vi "Read Test.vi"(8 "error in (no error)":errorcluster, 9 "data table":T1, 10 "data dictionary":refnum<class "data dictionary.lvclass">, 11 "runtime in":refnum<class "SystemLink File runtime.lvclass">) -> (0 "error out":errorcluster, 2 "Pass":bool[](array[boolean]), 3 "runtime out":refnum<class "SystemLink File runtime.lvclass">)   [LabVIEW 2015, in "SystemLink File Module tests.lvlib"]
uses:
  SystemLink File Module tests.lvlib
  <vilib>/NI/Tag Bus/dictionary/data dictionary.lvclass
  <vilib>/NI/Tag Bus/dictionary/lookup polymorphs/locate double.vi
  module/execution/SystemLink File runtime.lvclass
  <vilib>/NI/Tag Bus/table/data table.lvlib
  <vilib>/NI/Tag Bus/table/data polymorphs/read one/read Double.vi
  <vilib>/Skyline/Tag/Wrapper/Wrapper_class/NI Skyline Tag.lvclass
  <vilib>/Skyline/Tag/Wrapper/Wrapper AMQP_class/Open Tag AMQP.vi
  <vilib>/Skyline/Tag/Wrapper/Wrapper AMQP_class/NI Skyline Tag AMQP.lvclass
  <vilib>/Skyline/Tag/Wrapper/Wrapper_class/Write Tag (DBL).vi
  <vilib>/Skyline/Tag/Wrapper/Wrapper_class/Close Tag (Single).vi
  <vilib>/Skyline/Tag/Wrapper/Wrapper_class/Write Tag (I32).vi
  <vilib>/Skyline/Tag/Wrapper/Wrapper_class/Write Tag (String).vi
  <vilib>/NI/Tag Bus/table/data polymorphs/read one/read I32.vi
  <vilib>/NI/Tag Bus/dictionary/lookup polymorphs/locate I32.vi
  <vilib>/Skyline/Tag/Wrapper/Wrapper_class/Write Tag (U64).vi
  <vilib>/Skyline/Tag/Wrapper/Wrapper_class/Write Tag (Boolean).vi
  module/configuration/SystemLink File configuration.lvclass
  <vilib>/Skyline/Tag/Wrapper/Wrapper_class/Write Tag (Timestamp).vi
  <vilib>/NI/Tag Bus/dictionary/lookup polymorphs/locate Single.vi
  <vilib>/NI/Tag Bus/table/data polymorphs/read one/read Single.vi
  <vilib>/NI/Tag Bus/dictionary/lookup polymorphs/locate I16.vi
  <vilib>/NI/Tag Bus/table/data polymorphs/read one/read I16.vi
  <vilib>/NI/Tag Bus/dictionary/lookup polymorphs/locate I8.vi
  <vilib>/NI/Tag Bus/table/data polymorphs/read one/read I8.vi
  <vilib>/NI/Tag Bus/dictionary/lookup polymorphs/locate U64.vi
  <vilib>/NI/Tag Bus/table/data polymorphs/read one/read U64.vi
  <vilib>/NI/Tag Bus/dictionary/lookup polymorphs/locate U32.vi
  <vilib>/NI/Tag Bus/table/data polymorphs/read one/read U32.vi
  <vilib>/NI/Tag Bus/dictionary/lookup polymorphs/locate U16.vi
  <vilib>/NI/Tag Bus/table/data polymorphs/read one/read U16.vi
  <vilib>/NI/Tag Bus/dictionary/lookup polymorphs/locate U8.vi
  <vilib>/NI/Tag Bus/table/data polymorphs/read one/read U8.vi
  <vilib>/NI/Tag Bus/dictionary/lookup polymorphs/locate Boolean.vi
  <vilib>/NI/Tag Bus/table/data polymorphs/read one/read Boolean.vi
  <vilib>/NI/Tag Bus/dictionary/lookup polymorphs/locate String.vi
  <vilib>/NI/Tag Bus/table/data polymorphs/read one/read String.vi
  <vilib>/NI/Tag Bus/table/data table.ctl
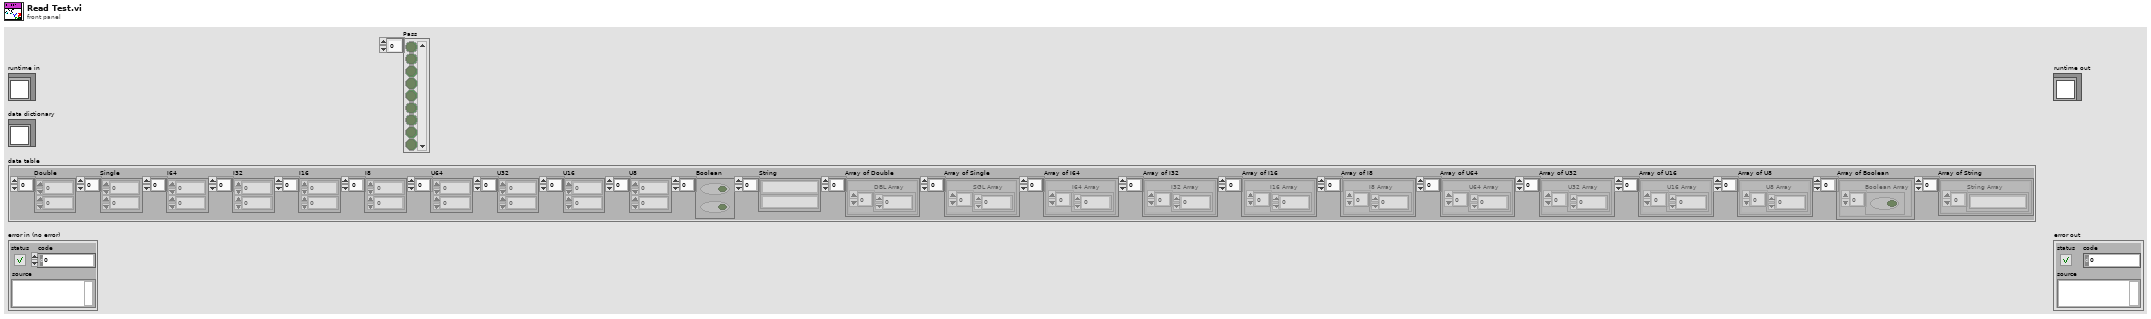
[diagram p1: front panel]
types:
  T1 = typedef "tag bus.lvlib/data table.lvlib/data table.ctl" = cluster{"Double":dbl[], "Single":sgl[], "I64":i64[], "I32":i32[], "I16":i16[], "I8":i8[], "U64":u64[], "U32":u32[], "U16":u16[], "U8":u8[], "Boolean":bool[], "String":string[], "Array of Double":cluster{"DBL Array":dbl[]}[], "Array of Single":cluster{"SGL Array":sgl[]}[], "Array of I64":cluster{"I64 Array":i64[]}[], "Array of I32":cluster{"I32 Array":i32[]}[], "Array of I16":cluster{"I16 Array":i16[]}[], "Array of I8":cluster{"I8 Array":i8[]}[], "Array of U64":cluster{"U64 Array":u64[]}[], "Array of U32":cluster{"U32 Array":u32[]}[], "Array of U16":cluster{"U16 Array":u16[]}[], "Array of U8":cluster{"U8 Array":u8[]}[], "Array of Boolean":cluster{"Boolean Array":bool[]}[], "Array of String":cluster{"String Array":string[]}[]}
  T2 = typedef "SystemLink File configuration.lvclass/SysLink Mapping.ctl" = cluster{"Data Type":T3, "Tag Reference":refnum<class "NI Skyline Tag.lvclass">, "Tag Bus Index":i32, "AMQP":bool, "Skylink Index":i32}
  T3 = typedef "SystemLink File configuration.lvclass/Data Tag Type.ctl" = enum16{"Double", "Single", "I32", "I16", "I8", "U64", "U32", "U16", "U8", "Boolean", "String", "Timestamp"}
  T4 = typedef "NI Skyline Tag.lvlib/DataType.ctl" = enum32{"Double", "I32", "String", "Boolean", "U64", "Timestamp"}
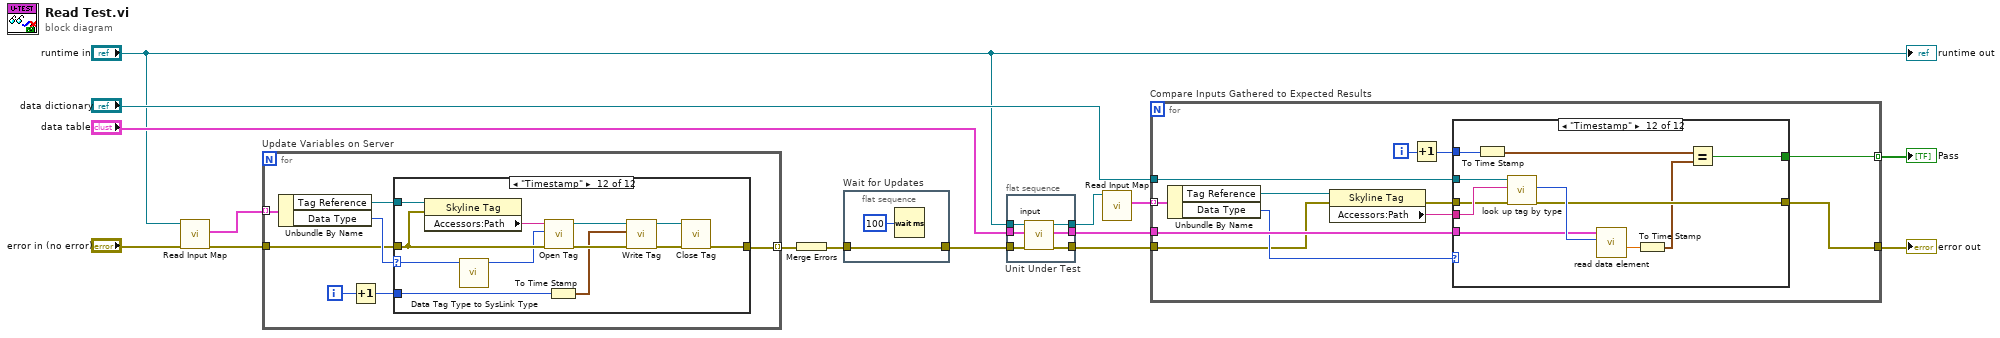
[diagram p0: block diagram]
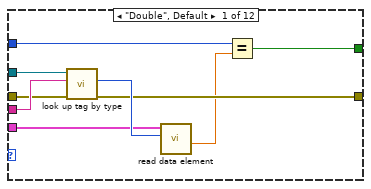
[diagram p2: hidden frame]
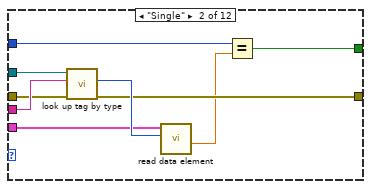
[diagram p3: hidden frame]
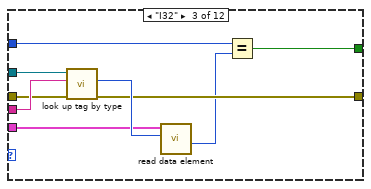
[diagram p4: hidden frame]
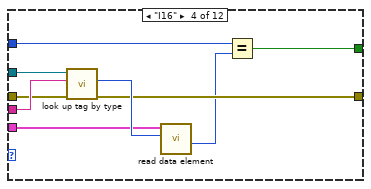
[diagram p5: hidden frame]
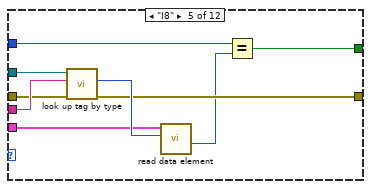
[diagram p6: hidden frame]
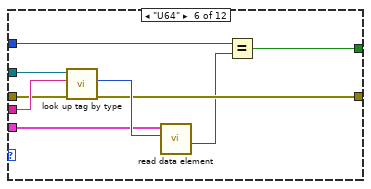
[diagram p7: hidden frame]
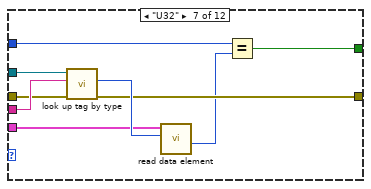
[diagram p8: hidden frame]
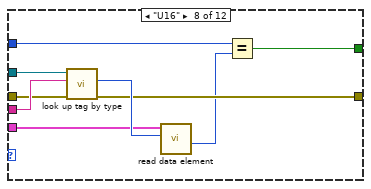
[diagram p9: hidden frame]
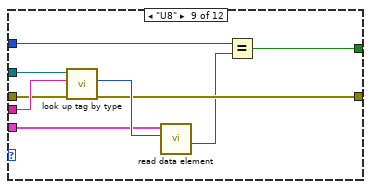
[diagram p10: hidden frame]
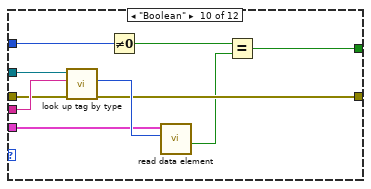
[diagram p11: hidden frame]
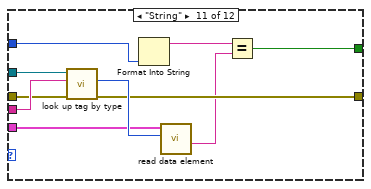
[diagram p12: hidden frame]
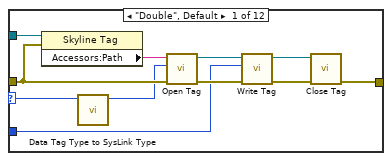
[diagram p13: hidden frame]
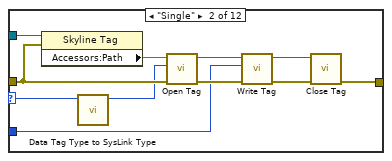
[diagram p14: hidden frame]
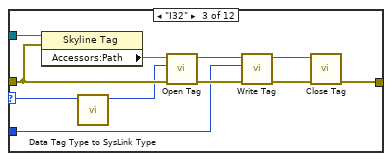
[diagram p15: hidden frame]
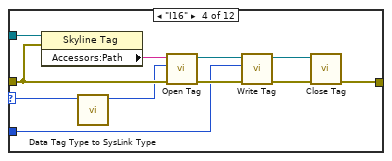
[diagram p16: hidden frame]
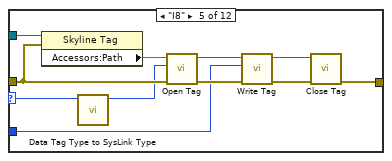
[diagram p17: hidden frame]
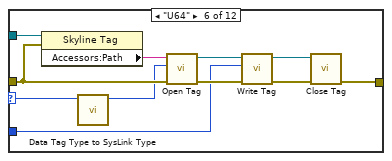
[diagram p18: hidden frame]
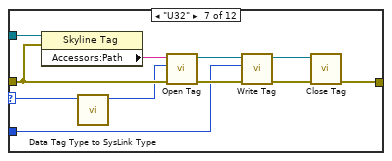
[diagram p19: hidden frame]
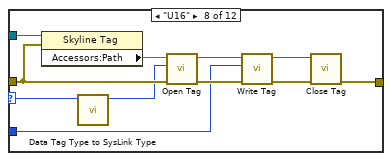
[diagram p20: hidden frame]
diagram:
  n1 = call "Read Input Map.vi"("error in (no error)"="error in (no error)", "SystemLink runtime in"="runtime in") -> ("error out"=w14:errorcluster, "Input Map"=w15:T2[])  [unwired: 7 in, 1 out]
  n2 = for "Update Variables on Server" {
    tunnel: w15 -> [w22] mode=indexing
    tunnel: w14 -> [w19]
    tunnel: [w16] -> w13 mode=indexing
    i -> [w18]
    n3 = Unbundle By Name(w22) -> ("Tag Reference"=w20:refnum<class "NI Skyline Tag.lvclass">, "Data Type"=w21:T3)
    n4 = Increment(x=w18) -> (x+1=w17:i32)
    n5 = case shown="\"Timestamp\"" w21 {
      selector: w21 -> [w30 w41 w52 w63 w74 w85 w96 w107 w118 w130 w142 w154]
      tunnel: w20 -> [w33 w44 w55 w66 w77 w88 w99 w110 w121 w133 w145 w157]
      tunnel: w19 -> [w31 w42 w53 w64 w75 w86 w97 w108 w119 w131 w143 w155]
      tunnel: w17 -> [w26 w37 w48 w59 w70 w81 w92 w103 w114 w126 w135 w147]
      tunnel: [w23 w34 w45 w56 w67 w78 w89 w100 w111 w123 w136 w148] -> w16
      frame "Double", Default {
        n6 = property class="Skyline Tag"(reference=w33, error in=w31) -> ("Accessors:Path"=w32:string)  [unwired: 2 out]
        n7 = call "Data Tag Type to SysLink Type.vi"("Data Tag Type"=w30) -> ("data type"=w29:T4)  [unwired: 10 in]
        n8 = call-poly <vilib>:"Open Tag.vi"("error in (no error)"=w31, "data type"=w29, "path"=w32) -> ("error out"=w27:errorcluster, "tag out"=w28:refnum<class "NI Skyline Tag.lvclass">)  [unwired: 7 in]
        n9 = call-poly <vilib>:"Write Tag.vi"("error in (no error)"=w27, "value"=w26, "tag in"=w28) -> ("error out"=w24:errorcluster, "tag out"=w25:refnum<class "NI Skyline Tag.lvclass">)  [unwired: 7 in]
        n10 = call-poly <vilib>:"Close Tag.vi"("error in (no error)"=w24, "tag in"=w25) -> ("error out"=w23:errorcluster)  [unwired: 9 in]
      }
      frame "Single" {
        n11 = property class="Skyline Tag"(reference=w44, error in=w42) -> ("Accessors:Path"=w43:string)  [unwired: 2 out]
        n12 = call "Data Tag Type to SysLink Type.vi"("Data Tag Type"=w41) -> ("data type"=w40:T4)  [unwired: 10 in]
        n13 = call-poly <vilib>:"Open Tag.vi"("error in (no error)"=w42, "data type"=w40, "path"=w43) -> ("error out"=w38:errorcluster, "tag out"=w39:refnum<class "NI Skyline Tag.lvclass">)  [unwired: 7 in]
        n14 = call-poly <vilib>:"Write Tag.vi"("error in (no error)"=w38, "value"=w37, "tag in"=w39) -> ("error out"=w35:errorcluster, "tag out"=w36:refnum<class "NI Skyline Tag.lvclass">)  [unwired: 7 in]
        n15 = call-poly <vilib>:"Close Tag.vi"("error in (no error)"=w35, "tag in"=w36) -> ("error out"=w34:errorcluster)  [unwired: 9 in]
      }
      frame "I32" {
        n16 = property class="Skyline Tag"(reference=w55, error in=w53) -> ("Accessors:Path"=w54:string)  [unwired: 2 out]
        n17 = call "Data Tag Type to SysLink Type.vi"("Data Tag Type"=w52) -> ("data type"=w51:T4)  [unwired: 10 in]
        n18 = call-poly <vilib>:"Open Tag.vi"("error in (no error)"=w53, "data type"=w51, "path"=w54) -> ("error out"=w49:errorcluster, "tag out"=w50:refnum<class "NI Skyline Tag.lvclass">)  [unwired: 7 in]
        n19 = call-poly <vilib>:"Write Tag.vi"("error in (no error)"=w49, "value"=w48, "tag in"=w50) -> ("error out"=w46:errorcluster, "tag out"=w47:refnum<class "NI Skyline Tag.lvclass">)  [unwired: 7 in]
        n20 = call-poly <vilib>:"Close Tag.vi"("error in (no error)"=w46, "tag in"=w47) -> ("error out"=w45:errorcluster)  [unwired: 9 in]
      }
      frame "I16" {
        n21 = property class="Skyline Tag"(reference=w66, error in=w64) -> ("Accessors:Path"=w65:string)  [unwired: 2 out]
        n22 = call "Data Tag Type to SysLink Type.vi"("Data Tag Type"=w63) -> ("data type"=w62:T4)  [unwired: 10 in]
        n23 = call-poly <vilib>:"Open Tag.vi"("error in (no error)"=w64, "data type"=w62, "path"=w65) -> ("error out"=w60:errorcluster, "tag out"=w61:refnum<class "NI Skyline Tag.lvclass">)  [unwired: 7 in]
        n24 = call-poly <vilib>:"Write Tag.vi"("error in (no error)"=w60, "value"=w59, "tag in"=w61) -> ("error out"=w57:errorcluster, "tag out"=w58:refnum<class "NI Skyline Tag.lvclass">)  [unwired: 7 in]
        n25 = call-poly <vilib>:"Close Tag.vi"("error in (no error)"=w57, "tag in"=w58) -> ("error out"=w56:errorcluster)  [unwired: 9 in]
      }
      frame "I8" {
        n26 = property class="Skyline Tag"(reference=w77, error in=w75) -> ("Accessors:Path"=w76:string)  [unwired: 2 out]
        n27 = call "Data Tag Type to SysLink Type.vi"("Data Tag Type"=w74) -> ("data type"=w73:T4)  [unwired: 10 in]
        n28 = call-poly <vilib>:"Open Tag.vi"("error in (no error)"=w75, "data type"=w73, "path"=w76) -> ("error out"=w71:errorcluster, "tag out"=w72:refnum<class "NI Skyline Tag.lvclass">)  [unwired: 7 in]
        n29 = call-poly <vilib>:"Write Tag.vi"("error in (no error)"=w71, "value"=w70, "tag in"=w72) -> ("error out"=w68:errorcluster, "tag out"=w69:refnum<class "NI Skyline Tag.lvclass">)  [unwired: 7 in]
        n30 = call-poly <vilib>:"Close Tag.vi"("error in (no error)"=w68, "tag in"=w69) -> ("error out"=w67:errorcluster)  [unwired: 9 in]
      }
      frame "U64" {
        n31 = property class="Skyline Tag"(reference=w88, error in=w86) -> ("Accessors:Path"=w87:string)  [unwired: 2 out]
        n32 = call "Data Tag Type to SysLink Type.vi"("Data Tag Type"=w85) -> ("data type"=w84:T4)  [unwired: 10 in]
        n33 = call-poly <vilib>:"Open Tag.vi"("error in (no error)"=w86, "data type"=w84, "path"=w87) -> ("error out"=w82:errorcluster, "tag out"=w83:refnum<class "NI Skyline Tag.lvclass">)  [unwired: 7 in]
        n34 = call-poly <vilib>:"Write Tag.vi"("error in (no error)"=w82, "value"=w81, "tag in"=w83) -> ("error out"=w79:errorcluster, "tag out"=w80:refnum<class "NI Skyline Tag.lvclass">)  [unwired: 7 in]
        n35 = call-poly <vilib>:"Close Tag.vi"("error in (no error)"=w79, "tag in"=w80) -> ("error out"=w78:errorcluster)  [unwired: 9 in]
      }
      frame "U32" {
        n36 = property class="Skyline Tag"(reference=w99, error in=w97) -> ("Accessors:Path"=w98:string)  [unwired: 2 out]
        n37 = call "Data Tag Type to SysLink Type.vi"("Data Tag Type"=w96) -> ("data type"=w95:T4)  [unwired: 10 in]
        n38 = call-poly <vilib>:"Open Tag.vi"("error in (no error)"=w97, "data type"=w95, "path"=w98) -> ("error out"=w93:errorcluster, "tag out"=w94:refnum<class "NI Skyline Tag.lvclass">)  [unwired: 7 in]
        n39 = call-poly <vilib>:"Write Tag.vi"("error in (no error)"=w93, "value"=w92, "tag in"=w94) -> ("error out"=w90:errorcluster, "tag out"=w91:refnum<class "NI Skyline Tag.lvclass">)  [unwired: 7 in]
        n40 = call-poly <vilib>:"Close Tag.vi"("error in (no error)"=w90, "tag in"=w91) -> ("error out"=w89:errorcluster)  [unwired: 9 in]
      }
      frame "U16" {
        n41 = property class="Skyline Tag"(reference=w110, error in=w108) -> ("Accessors:Path"=w109:string)  [unwired: 2 out]
        n42 = call "Data Tag Type to SysLink Type.vi"("Data Tag Type"=w107) -> ("data type"=w106:T4)  [unwired: 10 in]
        n43 = call-poly <vilib>:"Open Tag.vi"("error in (no error)"=w108, "data type"=w106, "path"=w109) -> ("error out"=w104:errorcluster, "tag out"=w105:refnum<class "NI Skyline Tag.lvclass">)  [unwired: 7 in]
        n44 = call-poly <vilib>:"Write Tag.vi"("error in (no error)"=w104, "value"=w103, "tag in"=w105) -> ("error out"=w101:errorcluster, "tag out"=w102:refnum<class "NI Skyline Tag.lvclass">)  [unwired: 7 in]
        n45 = call-poly <vilib>:"Close Tag.vi"("error in (no error)"=w101, "tag in"=w102) -> ("error out"=w100:errorcluster)  [unwired: 9 in]
      }
      frame "U8" {
        n46 = property class="Skyline Tag"(reference=w121, error in=w119) -> ("Accessors:Path"=w120:string)  [unwired: 2 out]
        n47 = call "Data Tag Type to SysLink Type.vi"("Data Tag Type"=w118) -> ("data type"=w117:T4)  [unwired: 10 in]
        n48 = call-poly <vilib>:"Open Tag.vi"("error in (no error)"=w119, "data type"=w117, "path"=w120) -> ("error out"=w115:errorcluster, "tag out"=w116:refnum<class "NI Skyline Tag.lvclass">)  [unwired: 7 in]
        n49 = call-poly <vilib>:"Write Tag.vi"("error in (no error)"=w115, "value"=w114, "tag in"=w116) -> ("error out"=w112:errorcluster, "tag out"=w113:refnum<class "NI Skyline Tag.lvclass">)  [unwired: 7 in]
        n50 = call-poly <vilib>:"Close Tag.vi"("error in (no error)"=w112, "tag in"=w113) -> ("error out"=w111:errorcluster)  [unwired: 9 in]
      }
      frame "Boolean" {
        n51 = property class="Skyline Tag"(reference=w133, error in=w131) -> ("Accessors:Path"=w132:string)  [unwired: 2 out]
        n52 = call "Data Tag Type to SysLink Type.vi"("Data Tag Type"=w130) -> ("data type"=w129:T4)  [unwired: 10 in]
        n53 = Not Equal To 0?(x=w126) -> (x != 0?=w122:bool)
        n54 = call-poly <vilib>:"Open Tag.vi"("error in (no error)"=w131, "data type"=w129, "path"=w132) -> ("error out"=w127:errorcluster, "tag out"=w128:refnum<class "NI Skyline Tag.lvclass">)  [unwired: 7 in]
        n55 = call-poly <vilib>:"Write Tag.vi"("error in (no error)"=w127, "value"=w122, "tag in"=w128) -> ("error out"=w124:errorcluster, "tag out"=w125:refnum<class "NI Skyline Tag.lvclass">)  [unwired: 7 in]
        n56 = call-poly <vilib>:"Close Tag.vi"("error in (no error)"=w124, "tag in"=w125) -> ("error out"=w123:errorcluster)  [unwired: 9 in]
      }
      frame "String" {
        n57 = property class="Skyline Tag"(reference=w145, error in=w143) -> ("Accessors:Path"=w144:string)  [unwired: 2 out]
        n58 = call "Data Tag Type to SysLink Type.vi"("Data Tag Type"=w142) -> ("data type"=w141:T4)  [unwired: 10 in]
        n59 = Format Into String(w135) -> (resulting string=w134:string)  [unwired: 3 in, 1 out]
        n60 = call-poly <vilib>:"Open Tag.vi"("error in (no error)"=w143, "data type"=w141, "path"=w144) -> ("error out"=w139:errorcluster, "tag out"=w140:refnum<class "NI Skyline Tag.lvclass">)  [unwired: 7 in]
        n61 = call-poly <vilib>:"Write Tag.vi"("error in (no error)"=w139, "value"=w134, "tag in"=w140) -> ("error out"=w137:errorcluster, "tag out"=w138:refnum<class "NI Skyline Tag.lvclass">)  [unwired: 7 in]
        n62 = call-poly <vilib>:"Close Tag.vi"("error in (no error)"=w137, "tag in"=w138) -> ("error out"=w136:errorcluster)  [unwired: 9 in]
      }
      frame "Timestamp" {
        n63 = property class="Skyline Tag"(reference=w157, error in=w155) -> ("Accessors:Path"=w156:string)  [unwired: 2 out]
        n64 = call "Data Tag Type to SysLink Type.vi"("Data Tag Type"=w154) -> ("data type"=w153:T4)  [unwired: 10 in]
        n65 = call-poly <vilib>:"Open Tag.vi"("error in (no error)"=w155, "data type"=w153, "path"=w156) -> ("error out"=w151:errorcluster, "tag out"=w152:refnum<class "NI Skyline Tag.lvclass">)  [unwired: 7 in]
        n66 = To Time Stamp(1:w147) -> (0:w146:timestamp)
        n67 = call-poly <vilib>:"Write Tag.vi"("error in (no error)"=w151, "value"=w146, "tag in"=w152) -> ("error out"=w149:errorcluster, "tag out"=w150:refnum<class "NI Skyline Tag.lvclass">)  [unwired: 7 in]
        n68 = call-poly <vilib>:"Close Tag.vi"("error in (no error)"=w149, "tag in"=w150) -> ("error out"=w148:errorcluster)  [unwired: 9 in]
      }
    }
  }
  n69 = Merge Errors(w13) -> (w12:errorcluster)
  n70 = flat-sequence "Wait for Updates" {
    tunnel: [w158] -> w10
    tunnel: w12 -> [w158]
    frame #0 {
      n71 = Wait (ms)(milliseconds to wait=u32 100) -> ()  [unwired: 1 out]
    }
  }
  n72 = flat-sequence "Unit Under Test" {
    tunnel: w10 -> [w165]
    tunnel: "runtime in" -> [w164]
    tunnel: "data table" -> [w163]
    tunnel: [w162] -> w8
    tunnel: [w161] -> w7
    tunnel: [w160] -> w5
    frame #0 {
      n73 = call-dynamic "input.vi"("error in"=w165, "input allocation"=w163, "module in"=w164) -> ("error out"=w161:errorcluster, "input data"=w160:T1, "module out"=w162:refnum<class "SystemLink File runtime.lvclass">)  [unwired: 6 in]
    }
  }
  n74 = call "Read Input Map.vi"("SystemLink runtime in"=w8) -> ("Input Map"=w6:T2[])  [unwired: 8 in, 2 out]
  n75 = for "Compare Inputs Gathered to Expected Results" {
    tunnel: w6 -> [w177] mode=indexing
    tunnel: w5 -> [w176]
    tunnel: "data dictionary" -> [w174]
    tunnel: w7 -> [w172]
    tunnel: [w167] -> w3
    tunnel: [w166] -> w2 mode=indexing
    i -> [w169]
    n76 = Unbundle By Name(w177) -> ("Tag Reference"=w173:refnum<class "NI Skyline Tag.lvclass">, "Data Type"=w175:T3)
    n77 = property class="Skyline Tag"(reference=w173, error in=w172) -> (error out=w171:errorcluster, "Accessors:Path"=w170:string)  [unwired: 1 out]
    n78 = Increment(x=w169) -> (x+1=w168:i32)
    n79 = case shown="\"Timestamp\"" w175 {
      tunnel: w171 -> [w184 w193 w202 w211 w220 w229 w238 w247 w256 w266 w276 w287]
      tunnel: w176 -> [w182 w191 w200 w209 w218 w227 w236 w245 w254 w264 w274 w285]
      tunnel: w174 -> [w186 w195 w204 w213 w222 w231 w240 w249 w258 w268 w278 w289]
      tunnel: w170 -> [w185 w194 w203 w212 w221 w230 w239 w248 w257 w267 w277 w288]
      tunnel: w168 -> [w179 w188 w197 w206 w215 w224 w233 w242 w251 w261 w269 w282]
      tunnel: [w181 w190 w199 w208 w217 w226 w235 w244 w253 w263 w273 w284] -> w167
      tunnel: [w178 w187 w196 w205 w214 w223 w232 w241 w250 w260 w271 w283] -> w166
      frame "Double", Default {
        n80 = call-poly <vilib>:"look up tag by type.vi"("error in"=w184, "name"=w185, "data dictionary in"=w186) -> ("error out"=w181:errorcluster, "index"=w183:i32)  [unwired: 6 in, 1 out]
        n81 = call-poly <vilib>:"read data element.vi"("index"=w183, "data table in"=w182) -> ("value"=w180:dbl)  [unwired: 8 in, 1 out]
        n82 = Equal?(x=w179, y=w180) -> (x = y?=w178:bool)
      }
      frame "Single" {
        n83 = call-poly <vilib>:"look up tag by type.vi"("error in"=w193, "name"=w194, "data dictionary in"=w195) -> ("error out"=w190:errorcluster, "index"=w192:i32)  [unwired: 6 in, 1 out]
        n84 = call-poly <vilib>:"read data element.vi"("index"=w192, "data table in"=w191) -> ("value"=w189:sgl)  [unwired: 8 in, 1 out]
        n85 = Equal?(x=w188, y=w189) -> (x = y?=w187:bool)
      }
      frame "I32" {
        n86 = call-poly <vilib>:"look up tag by type.vi"("error in"=w202, "name"=w203, "data dictionary in"=w204) -> ("error out"=w199:errorcluster, "index"=w201:i32)  [unwired: 6 in, 1 out]
        n87 = call-poly <vilib>:"read data element.vi"("index"=w201, "data table in"=w200) -> ("value"=w198:i32)  [unwired: 8 in, 1 out]
        n88 = Equal?(x=w197, y=w198) -> (x = y?=w196:bool)
      }
      frame "I16" {
        n89 = call-poly <vilib>:"look up tag by type.vi"("error in"=w211, "name"=w212, "data dictionary in"=w213) -> ("error out"=w208:errorcluster, "index"=w210:i32)  [unwired: 6 in, 1 out]
        n90 = call-poly <vilib>:"read data element.vi"("index"=w210, "data table in"=w209) -> ("value"=w207:i16)  [unwired: 8 in, 1 out]
        n91 = Equal?(x=w206, y=w207) -> (x = y?=w205:bool)
      }
      frame "I8" {
        n92 = call-poly <vilib>:"look up tag by type.vi"("error in"=w220, "name"=w221, "data dictionary in"=w222) -> ("error out"=w217:errorcluster, "index"=w219:i32)  [unwired: 6 in, 1 out]
        n93 = call-poly <vilib>:"read data element.vi"("index"=w219, "data table in"=w218) -> ("value"=w216:i8)  [unwired: 8 in, 1 out]
        n94 = Equal?(x=w215, y=w216) -> (x = y?=w214:bool)
      }
      frame "U64" {
        n95 = call-poly <vilib>:"look up tag by type.vi"("error in"=w229, "name"=w230, "data dictionary in"=w231) -> ("error out"=w226:errorcluster, "index"=w228:i32)  [unwired: 6 in, 1 out]
        n96 = call-poly <vilib>:"read data element.vi"("index"=w228, "data table in"=w227) -> ("value"=w225:u64)  [unwired: 8 in, 1 out]
        n97 = Equal?(x=w224, y=w225) -> (x = y?=w223:bool)
      }
      frame "U32" {
        n98 = call-poly <vilib>:"look up tag by type.vi"("error in"=w238, "name"=w239, "data dictionary in"=w240) -> ("error out"=w235:errorcluster, "index"=w237:i32)  [unwired: 6 in, 1 out]
        n99 = call-poly <vilib>:"read data element.vi"("index"=w237, "data table in"=w236) -> ("value"=w234:u32)  [unwired: 8 in, 1 out]
        n100 = Equal?(x=w233, y=w234) -> (x = y?=w232:bool)
      }
      frame "U16" {
        n101 = call-poly <vilib>:"look up tag by type.vi"("error in"=w247, "name"=w248, "data dictionary in"=w249) -> ("error out"=w244:errorcluster, "index"=w246:i32)  [unwired: 6 in, 1 out]
        n102 = call-poly <vilib>:"read data element.vi"("index"=w246, "data table in"=w245) -> ("value"=w243:u16)  [unwired: 8 in, 1 out]
        n103 = Equal?(x=w242, y=w243) -> (x = y?=w241:bool)
      }
      frame "U8" {
        n104 = call-poly <vilib>:"look up tag by type.vi"("error in"=w256, "name"=w257, "data dictionary in"=w258) -> ("error out"=w253:errorcluster, "index"=w255:i32)  [unwired: 6 in, 1 out]
        n105 = call-poly <vilib>:"read data element.vi"("index"=w255, "data table in"=w254) -> ("value"=w252:u8)  [unwired: 8 in, 1 out]
        n106 = Equal?(x=w251, y=w252) -> (x = y?=w250:bool)
      }
      frame "Boolean" {
        n107 = call-poly <vilib>:"look up tag by type.vi"("error in"=w266, "name"=w267, "data dictionary in"=w268) -> ("error out"=w263:errorcluster, "index"=w265:i32)  [unwired: 6 in, 1 out]
        n108 = Not Equal To 0?(x=w261) -> (x != 0?=w259:bool)
        n109 = call-poly <vilib>:"read data element.vi"("index"=w265, "data table in"=w264) -> ("value"=w262:bool)  [unwired: 8 in, 1 out]
        n110 = Equal?(x=w259, y=w262) -> (x = y?=w260:bool)
      }
      frame "String" {
        n111 = call-poly <vilib>:"look up tag by type.vi"("error in"=w276, "name"=w277, "data dictionary in"=w278) -> ("error out"=w273:errorcluster, "index"=w275:i32)  [unwired: 6 in, 1 out]
        n112 = Format Into String(w269) -> (resulting string=w270:string)  [unwired: 3 in, 1 out]
        n113 = call-poly <vilib>:"read data element.vi"("index"=w275, "data table in"=w274) -> ("value"=w272:string)  [unwired: 8 in, 1 out]
        n114 = Equal?(x=w270, y=w272) -> (x = y?=w271:bool)
      }
      frame "Timestamp" {
        n115 = To Time Stamp(1:w282) -> (0:w281:timestamp)
        n116 = call-poly <vilib>:"look up tag by type.vi"("error in"=w287, "name"=w288, "data dictionary in"=w289) -> ("error out"=w284:errorcluster, "index"=w286:i32)  [unwired: 6 in, 1 out]
        n117 = call-poly <vilib>:"read data element.vi"("index"=w286, "data table in"=w285) -> ("value"=w280:dbl)  [unwired: 8 in, 1 out]
        n118 = To Time Stamp(1:w280) -> (0:w279:timestamp)
        n119 = Equal?(x=w281, y=w279) -> (x = y?=w283:bool)
      }
    }
  }
  "error out" <- w3
  "Pass" <- w2
  "runtime out" <- "runtime in"
